vi "request fault.vi"(8 "error in":errorcluster, 9 "timeout in ms (0)":i32, 10 "rt fault":T1, 11 "worker comms in":T3) -> (0 "error out":errorcluster)   [LabVIEW 2013, in "worker pool.lvlib"]
uses:
  worker pool.lvlib
  worker comms.ctl
  worker commands.ctl
  request fifos.ctl
  recovery request.ctl
  <vilib>/NI/DCAF Module Framework/runtime/TBM module execution interface.lvclass
  <vilib>/NI/DCAF Module Framework/module configuration/TBM module configuration.lvclass
  rt fault.ctl
  <vilib>/NI/DCAF Module Framework/runtime/error classification.ctl
  response fifos.ctl
  recovery response.ctl
  <vilib>/NI/DCAF Execution Engine Interface/Engine Runtime/Fault.ctl
  <vilib>/NI/DCAF Execution Engine Interface/Engine Runtime/Engine Runtime Interface.lvclass
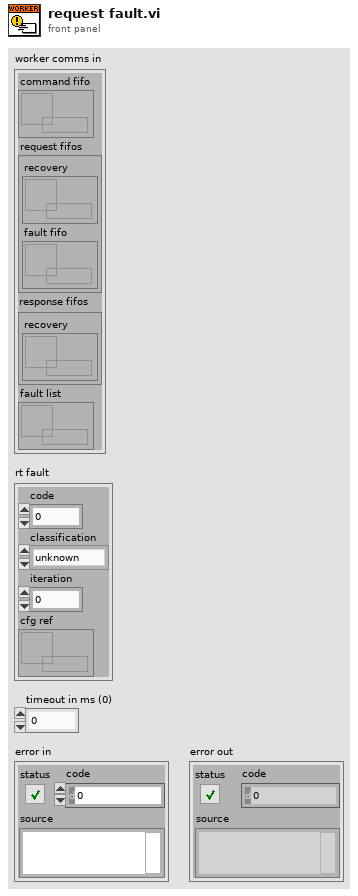
[diagram p1: front panel]
types:
  T1 = typedef "worker pool.lvlib/rt fault.ctl" = cluster{"code":i32, "classification":T2, "iteration":u64, "cfg ref":refnum<data-value>}
  T2 = typedef "TBM module execution interface.lvclass/error classification.ctl" = enum16{"unknown", "none", "trivial", "recoverable", "critical"}
  T3 = typedef "worker pool.lvlib/worker comms.ctl" = cluster{"command fifo":refnum<k33>, "request fifos":T4, "response fifos":T5, "fault list":refnum<data-value>}
  T4 = typedef "worker pool.lvlib/request fifos.ctl" = cluster{"recovery":refnum<k33>, "fault fifo":refnum<k33>}
  T5 = typedef "worker pool.lvlib/response fifos.ctl" = cluster{"recovery":refnum<k33>}
  T6 = typedef "worker pool.lvlib/worker commands.ctl" = enum16{"shutdown", "recover module", "record fault"}
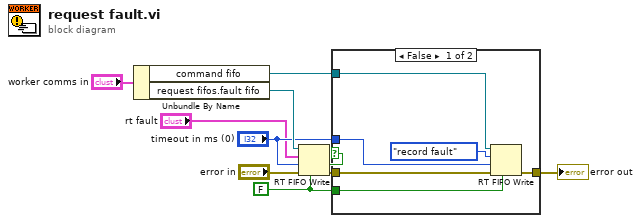
[diagram p0: block diagram]
diagram:
  w3 = FALSE ("overwrite on timeout (T)")
  n1 = Unbundle By Name("worker comms in") -> ("command fifo"=w5:refnum<k33>, "request fifos.fault fifo"=w6:refnum<k33>)
  n2 = RT FIFO Write(0:w6, 1:"rt fault", 2:"timeout in ms (0)", 3:"error in", 5:w3) -> (10:w4:bool, 11:w8:errorcluster)  [unwired: 2 out]
  n3 = case shown="False" w4 {
    tunnel: w8 -> [w16 w17]
    tunnel: [w15 w17] -> w7
    tunnel: w5 -> [w14 _]
    tunnel: w3 -> [w13 _]
    tunnel: "timeout in ms (0)" -> [w12 _]
    frame False {
      n4 = RT FIFO Write(0:w14, 1:worker_commands."record fault" ("element"), 2:w12, 3:w16, 5:w13) -> (11:w15:errorcluster)  [unwired: 3 out]
    }
    frame True {
    }
  }
  "error out" <- w7
